vi "PathPlanner_Path_CreatePath.vi"(9 "ConstraintZones":T5[](array[typedef]), 10 "HolonomicRotation":T6[](array[typedef]) {"target"."SIN" format="%13.4f"; "target"."COS" format="%13.4f"; "target"."VALUE" format="%13.4f"}, 11 "BezierPoints":T2[](array[typedef]) {"Y" format="%14.3f"; "X" format="%14.3f"}) -> (0 "Error":bool, 3 "Points":T1[](array[typedef]) {"HolonomicRotation"."SIN" format="%13.4f"; "HolonomicRotation"."COS" format="%13.4f"; "HolonomicRotation"."VALUE" format="%13.4f"; "Position"."Y" format="%14.3f"; "Position"."X" format="%14.3f"})   [LabVIEW 2019, in "PathPlanner24.lvlib"]
doc: "Create a path from an array of PathPlanner Waypoints. This routine calculates the trajectory states. It handles combining separate paths when reversal is flagged.\n\nInputs:\n - PathPlannerWaypoints -- An array of PathPlannerWaypoints. This array must contain at least 2 entries.\n - maxVel -- Max velocity of the path\n - maxAccel -- Max velocity of the path\n - reversed -- Should the robot follow the path reversed\n\nOutputs:\n - PathPlanner Trajectory -- The generated path (path planner trajectory) can be converted to trajectory)"
uses:
  PathPlanner24.lvlib
  <vilib>/Rock Robotics/WPI/ThirdParty/JAS_Junk/TrajLib/TypeDef/TRANSLATION2D.ctl
  TypeDef/PathPlannerRotationTarget.ctl
  <vilib>/Rock Robotics/WPI/ThirdParty/JAS_Junk/TrajLib/TypeDef/ROTATION2D.ctl
  TypeDef/PathPlannerConstraintsZone.ctl
  TypeDef/PathPlannerPathConstraints.ctl
  TypeDef/PathPlannerPathPoint.ctl
  PathPlanner_ConstraintsZone_GetAll.vi
  PathPlanner_ConstraintsZone_New.vi
  PathPlanner_RotationTarget_New.vi
  PathPlanner_PathSegment_Resolution.vi
  PathPlanner_PathSegment_FindConstraintZone.vi
  PathPlanner_PathPoint_New.vi
  PathPlanner_ConstraintsZone_IsWithinZone.vi
  PathPlanner_GeomUtil_CubicLerp.vi
  <vilib>/Rock Robotics/WPI/ThirdParty/JAS_Junk/TrajLib/Trajectory_Library.lvlib
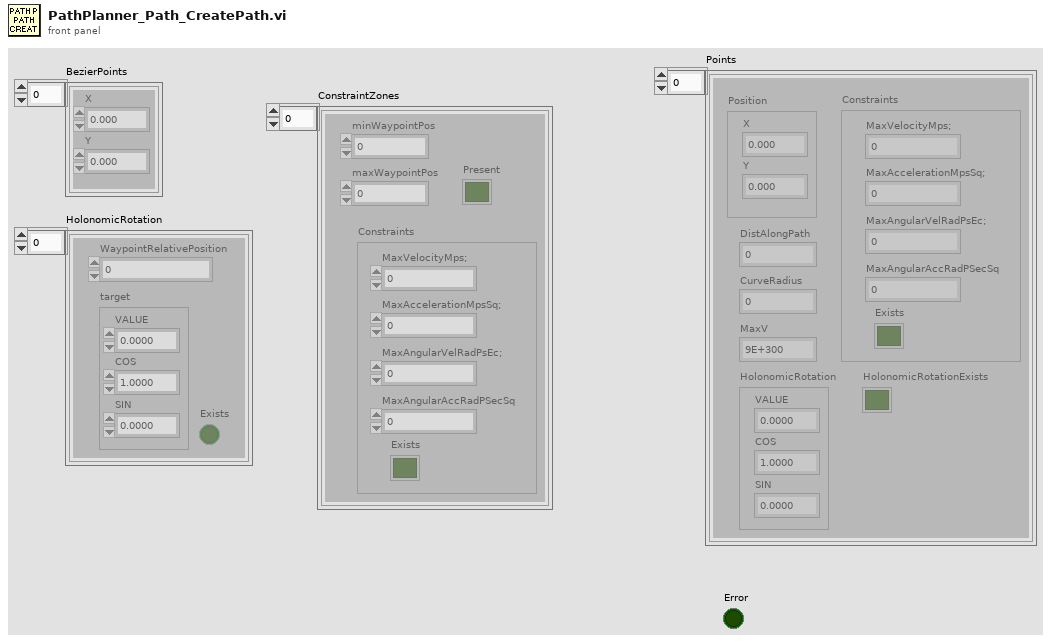
[diagram p1: front panel]
types:
  T1 = typedef "PathPlanner24.lvlib/PathPlannerPathPoint.ctl" = cluster{"Position":T2, "HolonomicRotation":T3, "DistAlongPath":dbl, "CurveRadius":dbl, "MaxV":dbl, "Constraints":T4, "HolonomicRotationExists":bool}
  T2 = typedef "Trajectory_Library.lvlib/TRANSLATION2D.ctl" = cluster{"X":dbl, "Y":dbl}
  T3 = typedef "Trajectory_Library.lvlib/ROTATION2D.ctl" = cluster{"VALUE":dbl, "COS":dbl, "SIN":dbl}
  T4 = typedef "PathPlanner24.lvlib/PathPlannerPathConstraints.ctl" = cluster{"MaxVelocityMps;":dbl, "MaxAccelerationMpsSq;":dbl, "MaxAngularVelRadPsEc;":dbl, "MaxAngularAccRadPSecSq":dbl, "Exists":bool}
  T5 = typedef "PathPlanner24.lvlib/PathPlannerConstraintsZone.ctl" = cluster{"minWaypointPos":dbl, "maxWaypointPos":dbl, "Constraints":T4, "Present":bool}
  T6 = typedef "PathPlanner24.lvlib/PathPlannerRotationTarget.ctl" = cluster{"target":T3, "WaypointRelativePosition":dbl, "Exists":bool}
  T7 = typedef "PathPlanner24.lvlib/PathPlannerPathSegment.ctl" = cluster{"SegmentPoints":T1[]}
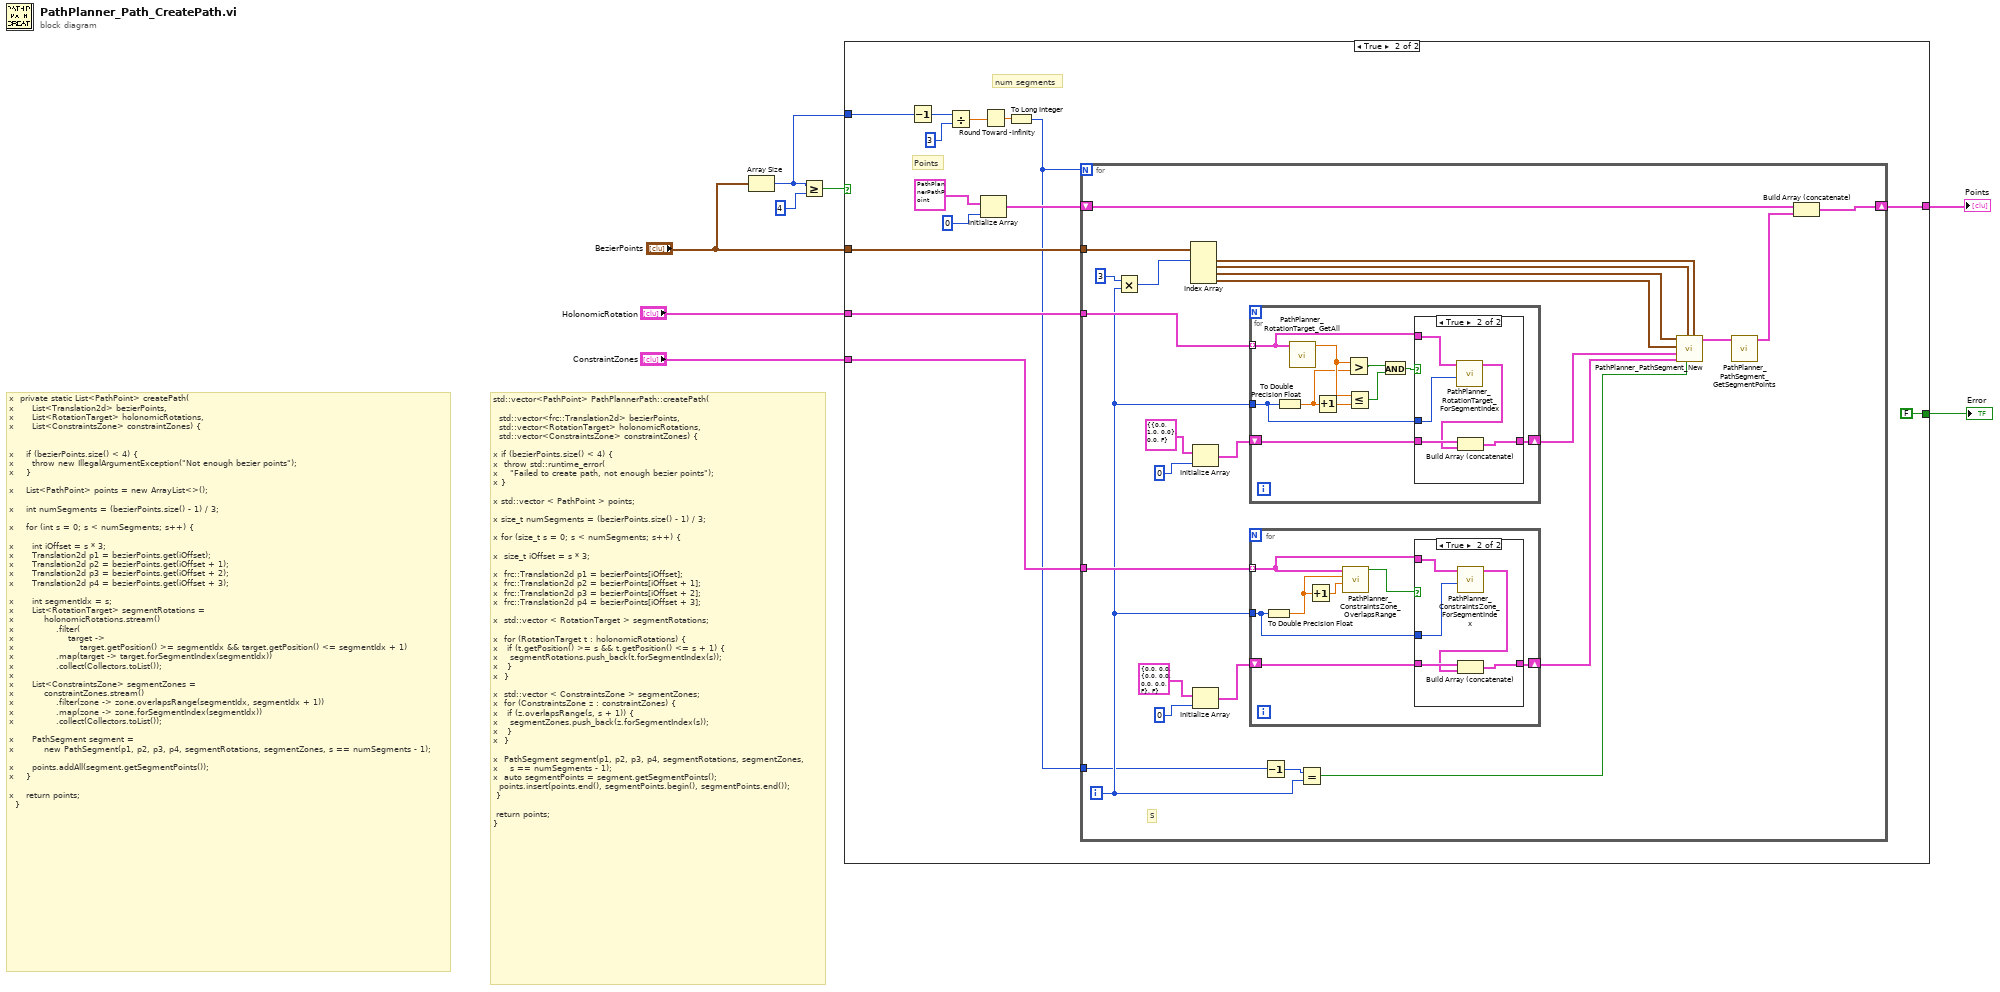
[diagram p0: block diagram]
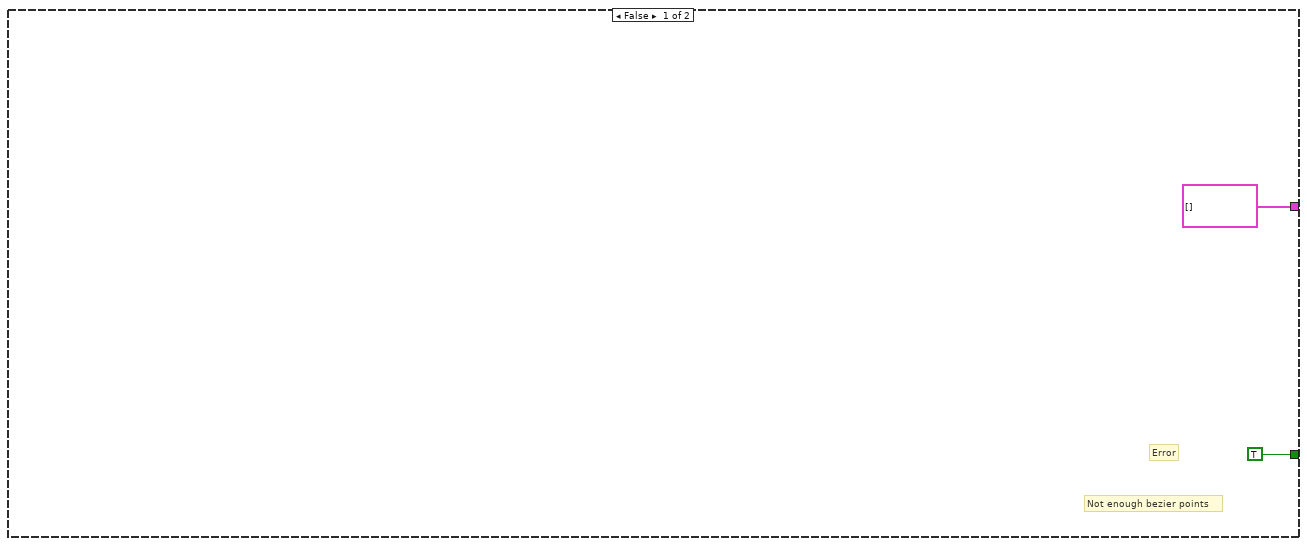
[diagram p2: hidden frame]
diagram:
  # "x  private static List<PathPoint> createPath(\nx      List<Translation2d> bezierPoints,\nx      List<RotationTarget> holonomicRotations,\nx      List<ConstraintsZone> constraintZones) {\n\n\nx    if (bezierPoints.size() < 4) {\nx      throw new IllegalArgumentException(\"Not enough bezier points\");\nx    }\n\nx    List<PathPoint> points = new ArrayList<>();\n\nx    int numSegments = (bezierPoints.size() - 1) / 3;\n\nx    for (int s = 0; s < numSegments; s++) {\n\nx      int iOffset = s * 3;\nx      Translation2d p1 = bezierPoints.get(iOffset);\nx      Translation2d p2 = bezierPoints.get(iOffset + 1);\nx      Translation2d p3 = bezierPoints.get(iOffset + 2);\nx      Translation2d p4 = bezierPoints.get(iOffset + 3);\n\nx      int segmentIdx = s;\nx      List<RotationTarget> segmentRotations =\nx          holonomicRotations.stream()\nx              .filter(\nx                  target ->\nx                      target.getPosition() >= segmentIdx && target.getPosition() <= segmentIdx + 1)\nx              .map(target -> target.forSegmentIndex(segmentIdx))\nx              .collect(Collectors.toList());\nx\nx      List<ConstraintsZone> segmentZones =\nx          constraintZones.stream()\nx              .filter(zone -> zone.overlapsRange(segmentIdx, segmentIdx + 1))\nx              .map(zone -> zone.forSegmentIndex(segmentIdx))\nx              .collect(Collectors.toList());\n\nx      PathSegment segment =\nx          new PathSegment(p1, p2, p3, p4, segmentRotations, segmentZones, s == numSegments - 1);\n\nx      points.addAll(segment.getSegmentPoints());\nx    }\n\nx    return points;\n  }"
  # "std::vector<PathPoint> PathPlannerPath::createPath(\n\n\t\tstd::vector<frc::Translation2d> bezierPoints,\n\t\tstd::vector<RotationTarget> holonomicRotations,\n\t\tstd::vector<ConstraintsZone> constraintZones) {\n\nx\tif (bezierPoints.size() < 4) {\nx\t\tthrow std::runtime_error(\nx\t\t\t\t\"Failed to create path, not enough bezier points\");\nx\t}\n\nx\tstd::vector < PathPoint > points;\n\nx\tsize_t numSegments = (bezierPoints.size() - 1) / 3;\n\t\nx for (size_t s = 0; s < numSegments; s++) {\n\nx\t\tsize_t iOffset = s * 3;\n\nx\t\tfrc::Translation2d p1 = bezierPoints[iOffset];\nx\t\tfrc::Translation2d p2 = bezierPoints[iOffset + 1];\nx\t\tfrc::Translation2d p3 = bezierPoints[iOffset + 2];\nx\t\tfrc::Translation2d p4 = bezierPoints[iOffset + 3];\n\nx\t\tstd::vector < RotationTarget > segmentRotations;\n\nx\t\tfor (RotationTarget t : holonomicRotations) {\nx\t\t\tif (t.getPosition() >= s && t.getPosition() <= s + 1) {\nx\t\t\t\tsegmentRotations.push_back(t.forSegmentIndex(s));\nx\t\t\t}\nx\t\t}\n\nx\t\tstd::vector < ConstraintsZone > segmentZones;\nx\t\tfor (ConstraintsZone z : constraintZones) {\nx\t\t\tif (z.overlapsRange(s, s + 1)) {\nx\t\t\t\tsegmentZones.push_back(z.forSegmentIndex(s));\nx\t\t\t}\nx\t\t}\n\nx\t\tPathSegment segment(p1, p2, p3, p4, segmentRotations, segmentZones,\nx\t\t\t\ts == numSegments - 1);\nx\t\tauto segmentPoints = segment.getSegmentPoints();\n\t\tpoints.insert(points.end(), segmentPoints.begin(), segmentPoints.end());\n\t}\n\n\treturn points;\n}"
  n1 = Array Size(array="BezierPoints") -> (size(s)=w4:i32)
  n2 = Greater Or Equal?(x=w4, y=4) -> (x >= y?=w7:bool)
  n3 = case shown="True" w7 {
    tunnel: [TRUE FALSE] -> w6
    tunnel: [T1[] [] ("Points") w11] -> w5
    tunnel: w4 -> [_ w21]
    tunnel: "BezierPoints" -> [_ w16]
    tunnel: "HolonomicRotation" -> [_ w15]
    tunnel: "ConstraintZones" -> [_ w14]
    frame False {
      # "Not enough bezier points"
      # "Error"
    }
    frame True {
      # "num segments"
      # "Points"
      n4 = Decrement(x=w21) -> (x-1=w20:i32)
      n5 = Divide(x=w20, y=3) -> (x/y=w18:dbl)
      n6 = Initialize Array(T1 {"Position"={"X"=0.0, "Y"=0.0}, "HolonomicRotation"={"VALUE"=0.0, "COS"=1.0, "SIN"=0.0}, "DistAlongPath"=0.0, "CurveRadius"=0.0, "MaxV"=9e+300, "Constraints"={"MaxVelocityMps;"=0.0, "MaxAccelerationMpsSq;"=0.0, "MaxAngularVelRadPsEc;"=0.0, "MaxAngularAccRadPSecSq"=0.0, "Exists"=FALSE}, "HolonomicRotationExists"=FALSE} ("PathPlannerPoint"), 0 ("dimension size")) -> (w23:T1[])
      n7 = Round Toward -Infinity(1:w18) -> (0:w17:dbl)
      n8 = To Long Integer(number=w17) -> (32bit integer=w13:i32)
      n9 = for {
        N: w13 -> [_]
        shift-right: [w25] -> w11
        shift-left: w23 -> [w27]
        tunnel: w16 -> [w47]
        tunnel: w15 -> [w46]
        tunnel: w14 -> [w39]
        tunnel: w13 -> [w31]
        i -> [w32]
        # "S"
        n10 = Multiply(x=3, y=w32) -> (x*y=w48:i32)
        n11 = Index Array(array=w47, index #1=w48) -> (element #1=w38:T2, element #2=w37:T2, element #3=w36:T2, element #4=w35:T2)  [unwired: 3 in]
        n12 = Initialize Array(T6 {"target"={"VALUE"=0.0, "COS"=1.0, "SIN"=0.0}, "WaypointRelativePosition"=0.0, "Exists"=FALSE} ("RotationTarget"), 0 ("dimension size")) -> (w43:T6[])
        n13 = Initialize Array(T5 {"minWaypointPos"=0.0, "maxWaypointPos"=0.0, "Constraints"={"MaxVelocityMps;"=0.0, "MaxAccelerationMpsSq;"=0.0, "MaxAngularVelRadPsEc;"=0.0, "MaxAngularAccRadPSecSq"=0.0, "Exists"=FALSE}, "Present"=FALSE} ("ConstraintsZone"), 0 ("dimension size")) -> (w40:T5[])
        n14 = for {
          tunnel: w46 -> [w66] mode=indexing
          tunnel: w32 -> [w63]
          shift-right: [w65] -> w34
          shift-left: w43 -> [w64]
          n15 = To Double Precision Float(number=w63) -> (double precision float=w69:dbl)
          n16 = call "PathPlanner_RotationTarget_GetAll.vi"("RotationTarget"=w66) -> ("WaypointRelativePosition"=w71:dbl)  [unwired: 9 in, 1 out]
          n17 = Increment(x=w69) -> (x+1=w70:dbl)
          n18 = Greater?(x=w71, y=w69) -> (0:w72:bool)
          n19 = Less Or Equal?(x=w71, y=w70) -> (x <= y?=w68:bool)
          n20 = And(x=w72, y=w68) -> (x .and. y?=w67:bool)
          n21 = case shown="True" w67 {
            tunnel: w66 -> [_ w76]
            tunnel: w64 -> [w73 w78]
            tunnel: [w73 w77] -> w65
            tunnel: w63 -> [_ w75]
            frame False {
            }
            frame True {
              n22 = call "PathPlanner_RotationTarget_ForSegmentIndex.vi"("SegmentIndex"=w75, "RotationTarget"=w76) -> ("new RotationTarget"=w74:T6)  [unwired: 9 in]
              n23 = Build Array (concatenate)(w78, w74) -> (w77:T6[])
            }
          }
        }
        n24 = for {
          tunnel: w39 -> [w54] mode=indexing
          tunnel: w32 -> [w50]
          shift-right: [w56] -> w33
          shift-left: w40 -> [w55]
          n25 = To Double Precision Float(number=w50) -> (double precision float=w53:dbl)
          n26 = Increment(x=w53) -> (x+1=w52:dbl)
          n27 = call "PathPlanner_ConstraintsZone_OverlapsRange.vi"("MaxPos"=w52, "MinPos"=w53, "ConstraintsZone"=w54) -> ("OverlapsRange"=w51:bool)  [unwired: 8 in]
          n28 = case shown="True" w51 {
            tunnel: w54 -> [_ w60]
            tunnel: w55 -> [w57 w62]
            tunnel: [w57 w61] -> w56
            tunnel: w50 -> [_ w59]
            frame False {
            }
            frame True {
              n29 = call "PathPlanner_ConstraintsZone_ForSegmentIndex.vi"("SegmentIndex"=w59, "ConstraintsZone"=w60) -> ("new Constraints Zone"=w58:T5)  [unwired: 9 in]
              n30 = Build Array (concatenate)(w62, w58) -> (w61:T5[])
            }
          }
        }
        n31 = Decrement(x=w31) -> (x-1=w30:i32)
        n32 = Equal?(x=w30, y=w32) -> (x = y?=w29:bool)
        n33 = call "PathPlanner_PathSegment_New.vi"("P1"=w38, "EndSegment"=w29, "P2"=w37, "ConstraintZones"=w33, "TargetHolonomicRotations"=w34, "P4"=w35, "P3"=w36) -> ("Segment"=w28:T7)  [unwired: 4 in]
        n34 = call "PathPlanner_PathSegment_GetSegmentPoints.vi"("Segment"=w28) -> ("SegmentPoints"=w26:T1[])  [unwired: 10 in]
        n35 = Build Array (concatenate)(w27, w26) -> (w25:T1[])
      }
    }
  }
  "Error" <- w6
  "Points" <- w5
